vi "SetupCLStim.vi"(0 "event port":u16=5557, 1 "OEP pulse channel":u16=2 caption="probe channel" min=1 max=8, 2 "Analog pulse channel":tag="pciDAQ/ao0", 3 "Digital real/sham stim channels":tag="pciDAQ/port0/line1:2", 4 "OEP sample clock in":tag="/pciDAQ/PFI0", 5 "Onboard counter":tag="pciDAQ/ctr0") -> (9 "zmq error out":errorcluster, 10 "context out":refnum<class "zmq_context.lvclass">, 11 "socket out":refnum<class "zmq_socket.lvclass">, 13 "clock offset":i64, 14 "AO task out":refnum<k21>, 15 "AO error out":errorcluster, 16 "DO task out":refnum<k21>, 17 "DO error out":errorcluster, 18 "ctr task out":refnum<k21>, 19 "ctr error out":errorcluster)   [LabVIEW 2017]
uses:
  <vilib>/addons/zeromq/zmq_socket.lvclass
  <vilib>/addons/zeromq/zmq_context.lvclass
  <vilib>/DAQmx/write.llb/DAQmx Write (Digital 1D Bool 1Chan 1Samp).vi
  <vilib>/DAQmx/read.llb/DAQmx Read (Counter U32 1Chan 1Samp).vi
  <vilib>/DAQmx/miscellaneous.llb/DAQmx Fill In Error Info.vi
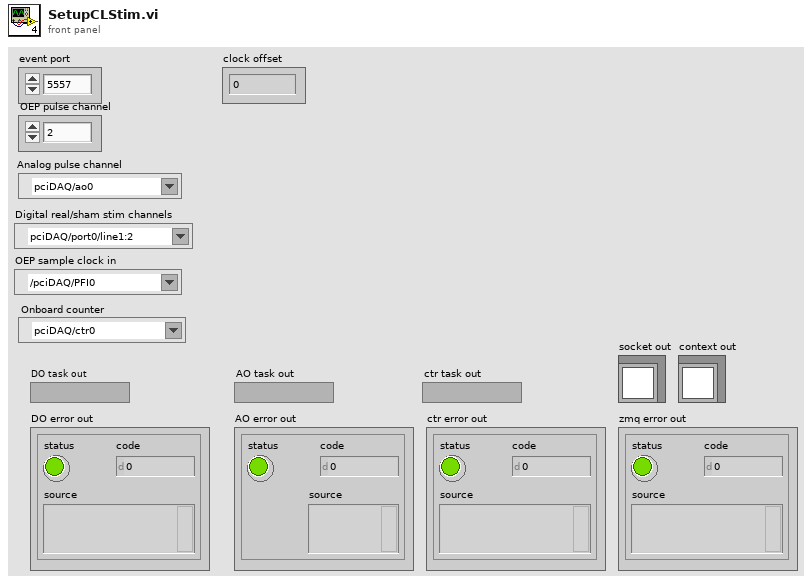
[diagram p1: front panel]
types:
  T1 = typedef "Rendezvous RefNum" = refnum<k1>
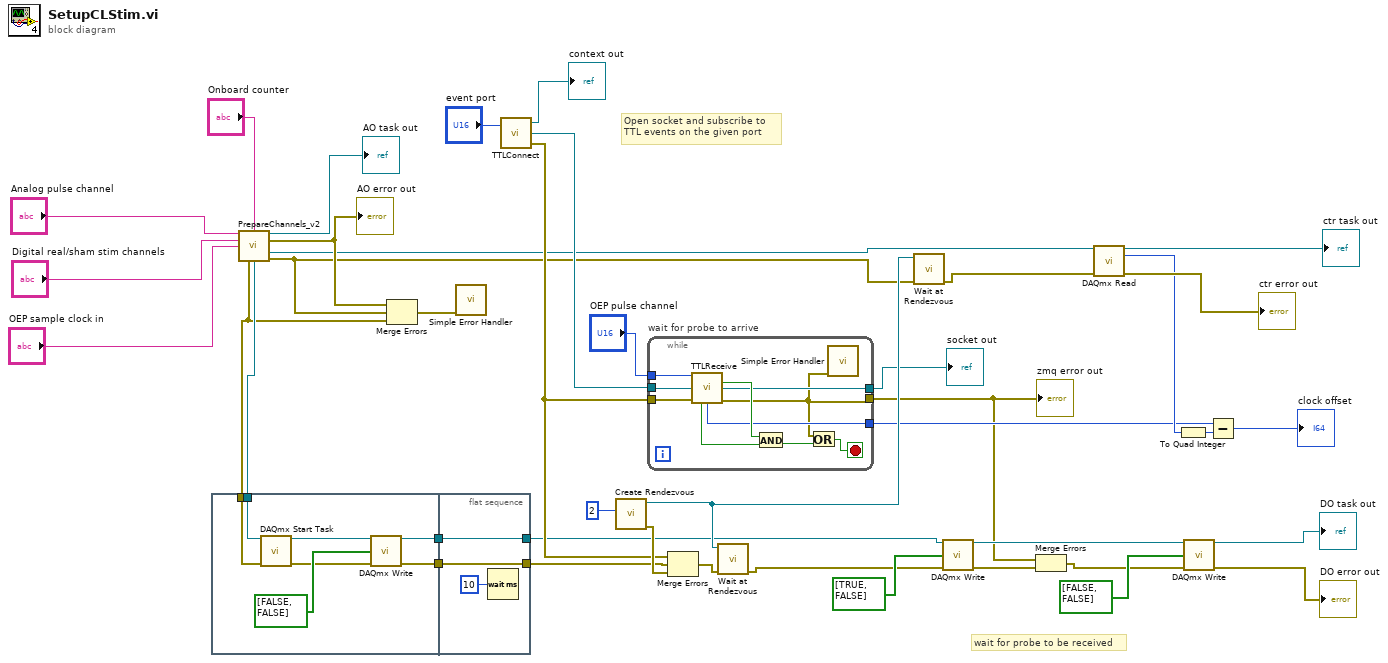
[diagram p0: block diagram]
diagram:
  # "wait for probe to be received"
  # "Open socket and subscribe to\nTTL events on the given port"
  n1 = flat-sequence {
    tunnel: w5 -> [w48]
    tunnel: w8 -> [w47]
    tunnel: [w43] -> w4
    tunnel: [w42] -> w2
    tunnel: [w50] -> w3
    tunnel: w4 -> [w50]
    tunnel: [w49] -> w1
    tunnel: w2 -> [w49]
    frame #0 {
      n2 = call <vilib>:"DAQmx Start Task.vi"("task/channels in"=w47, "error in"=w48) -> ("task out"=w45:refnum<k21>, "error out"=w44:errorcluster)  [unwired: 12 in]
      n3 = call-poly <vilib>:"DAQmx Write.vi"("task/channels in"=w45, "data"=bool[] [FALSE, FALSE], "error in"=w44) -> ("task out"=w42:refnum<k21>, "error out"=w43:errorcluster)  [unwired: 10 in, 1 out]
    }
    frame #1 {
      n4 = Wait (ms)(milliseconds to wait=u32 10) -> ()  [unwired: 1 out]
    }
  }
  n5 = call "PrepareChannels_v2.vi"("AO Physical channels"="Analog pulse channel", "Onboard counter"="Onboard counter", "DO Physical channels"="Digital real/sham stim channels", "OEP sample clock in"="OEP sample clock in") -> ("AO task out"=→"AO task out":refnum<k21>, "AO error out"=w39:errorcluster, "ctr task out"=w7:refnum<k21>, "DO error out"=w5:errorcluster, "DO task out"=w8:refnum<k21>, "ctr error out"=w6:errorcluster)  [unwired: 5 in, 1 out]
  "AO error out" <- w39
  n6 = Merge Errors(w39, w6, w5) -> (w38:errorcluster)
  n7 = call <vilib>:"Simple Error Handler.vi"("error in (no error)"=w38) -> ()  [unwired: 4 in, 5 out]
  n8 = call "TTLConnect.vi"("port"="event port") -> ("context out"=→"context out":refnum<class "zmq_context.lvclass">, "socket out"=w15:refnum<class "zmq_socket.lvclass">, "error out"=w25:errorcluster)  [unwired: 1 in]
  n9 = call <vilib>:"Create Rendezvous.vi"("size (2)"=2) -> ("error out"=w30:errorcluster, "rendezvous"=w26:T1)  [unwired: 4 in, 1 out]
  n10 = while "wait for probe to arrive" {
    tunnel: w15 -> [w61]
    tunnel: "OEP pulse channel" -> [w60]
    tunnel: [w57] -> w17
    tunnel: [w52] -> w9
    tunnel: [w56] -> w19
    tunnel: w25 -> [w55]
    stop <- w54 stop-if-true
    n11 = call "TTLReceive.vi"("channel"=w60, "socket in"=w61, "error in"=w55) -> ("new TTL"=w59:bool, "socket out"=w56:refnum<class "zmq_socket.lvclass">, "event on"=w58:bool, "timestamp"=w57:i64, "error out"=w52:errorcluster)  [unwired: 7 in, 1 out]
    n12 = And(x=w59, y=w58) -> (x .and. y?=w53:bool)
    n13 = Or(x=w52, y=w53) -> (x .or. y?=w54:bool)
    n14 = call <vilib>:"Simple Error Handler.vi"("error in (no error)"=w52) -> ()  [unwired: 4 in, 5 out]
  }
  "zmq error out" <- w9
  "socket out" <- w19
  n15 = Merge Errors(w25, w3, w30) -> (w27:errorcluster)
  n16 = call <vilib>:"Wait at Rendezvous.vi"("error in (no error)"=w27, "rendezvous"=w26) -> ("error out"=w28:errorcluster)  [unwired: 3 in, 2 out]
  n17 = call <vilib>:"Wait at Rendezvous.vi"("error in (no error)"=w6, "rendezvous"=w26) -> ("error out"=w24:errorcluster)  [unwired: 3 in, 2 out]
  n18 = call-poly <vilib>:"DAQmx Write.vi"("task/channels in"=w1, "data"=bool[] [TRUE, FALSE], "error in"=w28) -> ("task out"=w21:refnum<k21>, "error out"=w11:errorcluster)  [unwired: 10 in, 1 out]
  n19 = Merge Errors(w9, w11) -> (w10:errorcluster)
  n20 = call-poly <vilib>:"DAQmx Read.vi"("task/channels in"=w7, "error in"=w24) -> ("task out"=→"ctr task out":refnum<k21>, "data"=w22:u32, "error out"=→"ctr error out":errorcluster)  [unwired: 11 in]
  n21 = To Quad Integer(1:w22) -> (0:w20:i64)
  n22 = call-poly <vilib>:"DAQmx Write.vi"("task/channels in"=w21, "data"=bool[] [FALSE, FALSE], "error in"=w10) -> ("task out"=→"DO task out":refnum<k21>, "error out"=→"DO error out":errorcluster)  [unwired: 10 in, 1 out]
  n23 = Subtract(x=w17, y=w20) -> (x-y=→"clock offset":i64)
